vi "EditOptions.vi"(8 "error in":errorcluster, 11 "node in":refnum<class "My System.lvclass">) -> (0 "error out":errorcluster, 1 "edit options":T1, 2 "subnodes class":T2, 3 "node out":refnum<class "My System.lvclass">)   [LabVIEW 2014, in "My System.lvclass"]
doc: "Contains the options for the Menu that will be displayed when doing right click on an item.\nThe sub nodes class configures which nodes can be added to this nodes\nAnd the edit options determine which options are available for the node.\nThis configuration is stored in this VI in case some dynamic configuration is required for the menu options or sub nodes."
uses:
  My System.lvclass
  <vilib>/NI/Configuration Framework/Node/SubNodeCluster.ctl
  <vilib>/NI/Configuration Framework/Node/NodeMenuOptions.ctl
  <vilib>/NI/Configuration Framework/Node/NISE_CEF_Node.lvclass
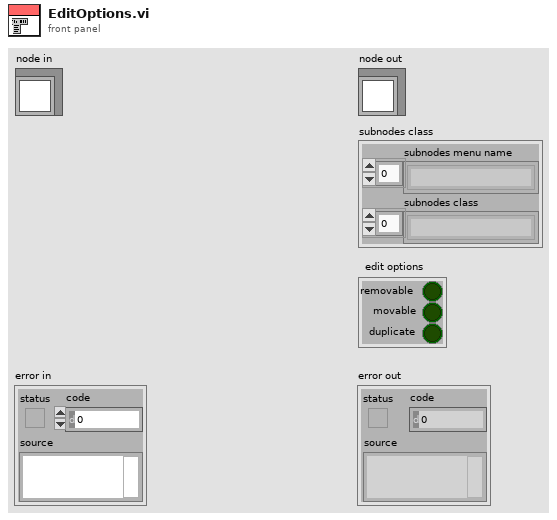
[diagram p1: front panel]
types:
  T1 = typedef "NISE_CEF_Node.lvclass/NodeMenuOptions.ctl" = cluster{"removable":bool, "movable":bool, "duplicate":bool}
  T2 = typedef "NISE_CEF_Node.lvclass/SubNodeCluster.ctl" = cluster{"subnodes menu name":string[], "subnodes class":string[]}
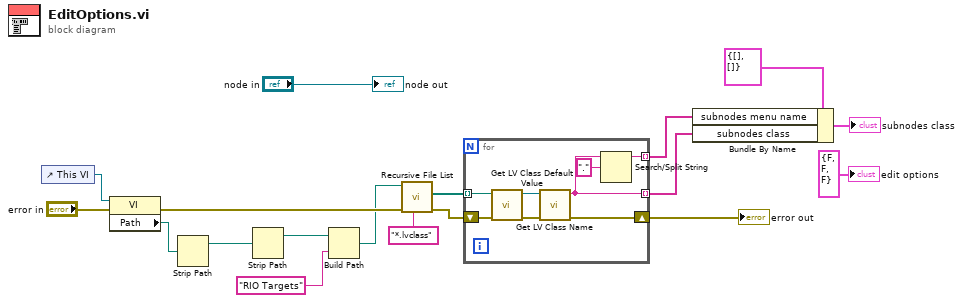
[diagram p0: block diagram]
diagram:
  n1 = control-ref of="This VI"() -> (w12:refnum<vi>)
  n2 = property class="VI"(reference=w12, error in="error in") -> (error out=w11:errorcluster, "Path"=w14:path)  [unwired: 1 out]
  n3 = Strip Path(path=w14) -> (stripped path=w9:path)  [unwired: 1 out]
  n4 = Strip Path(path=w9) -> (stripped path=w8:path)  [unwired: 1 out]
  n5 = Build Path(base path=w8, name or relative path="RIO Targets") -> (appended path=w10:path)
  n6 = call <vilib>:"Recursive File List.vi"("pattern"="*.lvclass", "error in (no error)"=w11, "Folder Path"=w10) -> ("error out"=w16:errorcluster, "All Files in Dir"=w17:path[])  [unwired: 4 in, 3 out]
  n7 = for {
    tunnel: w17 -> [w24] mode=indexing
    shift-right: [w22] -> w1
    shift-left: w16 -> [w23]
    tunnel: [w20] -> w5 mode=indexing
    tunnel: [w19] -> w6 mode=indexing
    n8 = call <vilib>:"Get LV Class Default Value.vi"("error in (no error)"=w23, "class path"=w24) -> ("error out"=w25:errorcluster, "object"=w26:refnum<class>)  [unwired: 8 in]
    n9 = call <vilib>:"Get LV Class Name.vi"("error in (no error)"=w25, "object"=w26) -> ("error out"=w22:errorcluster, "class name"=w20:string)  [unwired: 8 in]
    n10 = Search/Split String(string=w20, search string/char (-)=".") -> (substring before match=w19:string)  [unwired: 1 in, 2 out]
  }
  "error out" <- w1
  n11 = Bundle By Name(cluster=T2 {"subnodes menu name"=[], "subnodes class"=[]} ("subnodes class"), "subnodes menu name"=w6, "subnodes class"=w5) -> (→"subnodes class":T2)
  "node out" <- "node in"
  "edit options" <- T1 {"removable"=FALSE, "movable"=FALSE, "duplicate"=FALSE} ("edit options")
